vi "niHWS Set Scaling Coefficients.vi"(8 "error in (no error)":errorcluster, 10 "coefficient array":dbl[](array[numeric]) format="%0.2f", 11 "waveform reference in":u32) -> (0 "error out":errorcluster, 3 "waveform reference out":u32)   [LabVIEW 2013]
doc: "Establishes an Nth degree polynomial scaling function.\n\nWhen an analog waveform stored as integer data is retrieved by a floating-point read or retrieve function, NI-HWS scales the data according to this polynomial scaling function."
uses:
  nihwsu.dll
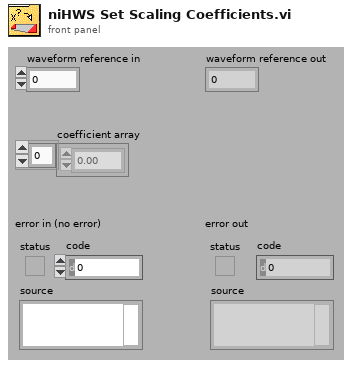
[diagram p1: front panel]
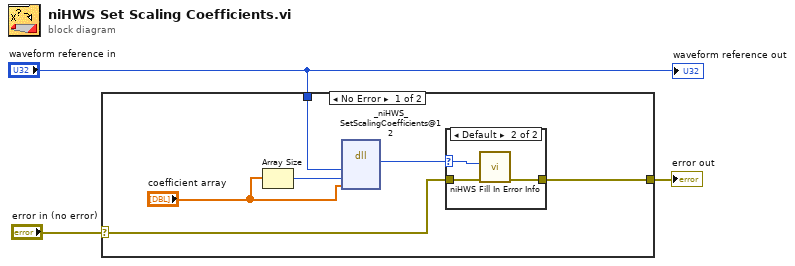
[diagram p0: block diagram]
diagram:
  n1 = case shown="No Error" "error in (no error)" {
    selector: "error in (no error)" -> [w5 w14]
    tunnel: [w6 w14] -> w2
    tunnel: "waveform reference in" -> [w7 _]
    frame No Error {
      n2 = Array Size(array="coefficient array") -> (size(s)=w8:i32)
      n3 = dll-call lib="nihwsu.dll" fn="_niHWS_SetScalingCoefficients@12"("wfmReference"=w7, "numCoeffs"=w8, "coeffArray"="coefficient array") -> (w4:i32)  [unwired: 6 in, 2 out]
      n4 = case shown="Default" w4 {
        selector: w4 -> [_ w11]
        tunnel: [w10 w12] -> w6
        tunnel: w5 -> [w10 w13]
        frame 0 {
        }
        frame Default {
          n5 = call "niHWS Fill In Error Info.vi"("error in (no error)"=w13, "status code"=w11) -> ("error out"=w12:errorcluster)  [unwired: 9 in]
        }
      }
    }
    frame Error {
    }
  }
  "error out" <- w2
  "waveform reference out" <- "waveform reference in"
